vi "Wait For Write Space.vi"(8 "error in (no error)":errorcluster, 9 "BufferSize":i32, 10 "timeout (ms)":i32=5000, 11 "AO Tasks":T1[](array[typedef])) -> (0 "error out":errorcluster={"status"=FALSE, "code"=555, "source"="Timed out waiting for Signal Bank."}, 2 "Timeout (ms)":i32, 3 "SpaceAvail":u32)   [LabVIEW 2020]
uses:
  Type Defs/Task Struct.ctl
  PXI Globals.vi
  <resource>/objmgr/daqmx.rc
panel:
  out "Time (ms)":u32
  out "SpaceAvail":u32
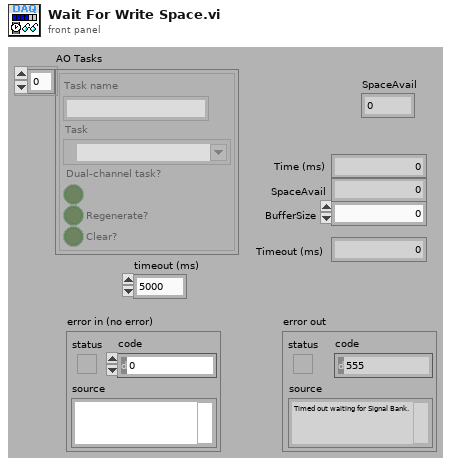
[diagram p1: front panel]
types:
  T1 = typedef "Task Struct.ctl" = cluster{"Task name":string, "Task":refnum<k21>, "Dual-channel task?":bool, "Regenerate?":bool, "Clear?":bool}
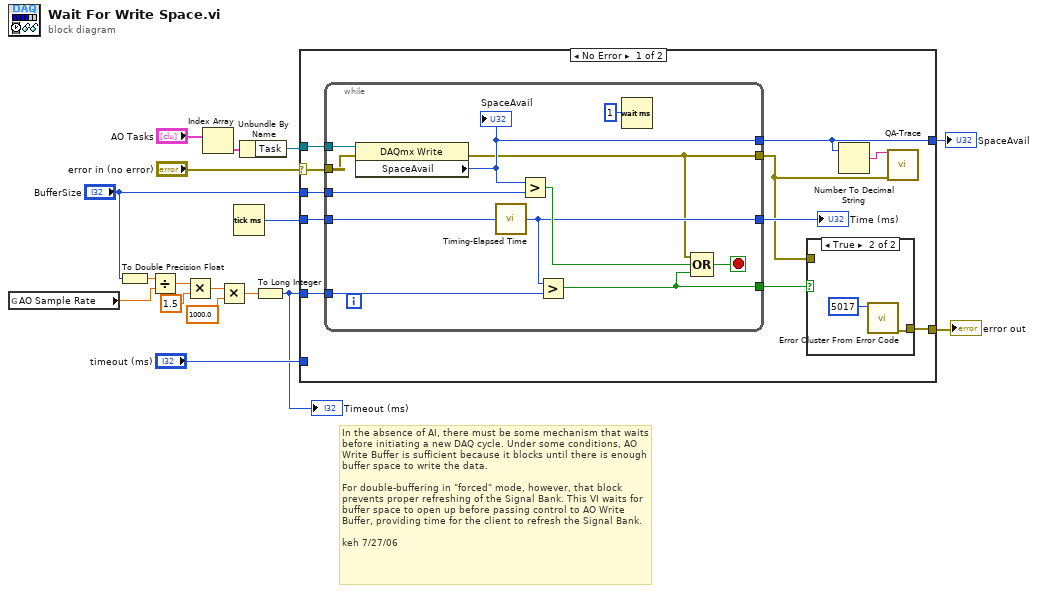
[diagram p0: block diagram]
diagram:
  # "In the absence of AI, there must be some mechanism that waits before initiating a new DAQ cycle. Under some conditions, AO Write Buffer is sufficient because it blocks until there is enough buffer space to write the data.\n\nFor double-buffering in \"forced\" mode, however, that block prevents proper refreshing of the Signal Bank. This VI waits for buffer space to open up before passing control to AO Write Buffer, providing time for the client to refresh the Signal Bank.\n\nkeh 7/27/06"
  n1 = global read "PXI Globals.vi" "AO Sample Rate"() -> (w9:dbl)
  n2 = To Double Precision Float(number="BufferSize") -> (double precision float=w11:dbl)
  n3 = Divide(x=w11, y=w9) -> (x/y=w8:dbl)
  n4 = Multiply(x=w8, y=1.5) -> (x*y=w6:dbl)
  n5 = Index Array(array="AO Tasks") -> (element=w15:T1)  [unwired: 1 in]
  n6 = Multiply(x=w6, y=1000.0) -> (x*y=w4:dbl)
  n7 = Tick Count (ms)() -> (millisecond timer value=w2:u32)
  n8 = Unbundle By Name(w15) -> ("Task"=w14:refnum<k21>)
  n9 = To Long Integer(number=w4) -> (32bit integer=w3:i32)
  "Timeout (ms)" <- w3
  n10 = case shown="No Error" "error in (no error)" {
    selector: "error in (no error)" -> [w25 w44]
    tunnel: "timeout (ms)" -> [_ _]
    tunnel: w14 -> [w27 _]
    tunnel: "BufferSize" -> [w26 _]
    tunnel: [w28 w44] -> w12
    tunnel: w2 -> [w23 _]
    tunnel: w3 -> [w24 _]
    tunnel: [w19 _] -> w1
    frame No Error {
      n11 = while {
        tunnel: [w41] -> w18
        tunnel: w27 -> [w33]
        tunnel: w25 -> [w38]
        tunnel: [w32] -> w21
        tunnel: w26 -> [w40]
        tunnel: w23 -> [w36]
        tunnel: w24 -> [w39]
        tunnel: [w35] -> w22
        tunnel: [w34] -> w19
        stop <- w42 stop-if-true
        n12 = property class="DAQmx Write"(reference=w33, error in=w38) -> (error out=w32:errorcluster, "SpaceAvail"=w34:u32)  [unwired: 1 out]
        "SpaceAvail" <- w34
        n13 = call "Timing-Elapsed Time.vi"("Start time (ms)"=w36) -> ("Elapsed time (ms)"=w35:u32)  [unwired: 4 in]
        n14 = Greater?(x=w34, y=w40) -> (0:w37:bool)
        n15 = Greater?(x=w35, y=w39) -> (0:w41:bool)
        n16 = Wait (ms)(milliseconds to wait=1) -> ()  [unwired: 1 out]
        n17 = Compound Arithmetic op=OR(w32, w37, w41) -> (w42:bool)
      }
      "Time (ms)" <- w22
      n18 = case shown="True" w18 {
        tunnel: [w29 w31] -> w28
        tunnel: w21 -> [w29 _]
        frame False {
        }
        frame True {
          n19 = call <vilib>:"Error Cluster From Error Code.vi"("error code (0)"=5017) -> ("error out"=w31:errorcluster)  [unwired: 8 in]
        }
      }
      n20 = Number To Decimal String(number=w19) -> (decimal integer string=w20:string)  [unwired: 1 in]
      n21 = call "QA-Trace.vi"("trace string"=w20, "error in (no error)"=w21) -> ()  [unwired: 13 in, 1 out]
    }
    frame Error {
    }
  }
  "error out" <- w12
  "SpaceAvail" <- w1
